vi "Read Enabled Values.vi"(8 "error in (no error)":errorcluster, 11 "No-Op in":refnum<class "No-Op Output.lvclass">) -> (0 "error out":errorcluster, 1 "Data Values Native":dbl[](array[numeric]), 2 "Data Values Engineering":dbl[](array[numeric]), 3 "No-Op out":refnum<class "No-Op Output.lvclass">)   [LabVIEW 2018, in "No-Op Output.lvclass"]
uses:
  No-Op Output.lvclass
  No-Op Output.lvclass/No-Op Output.ctl
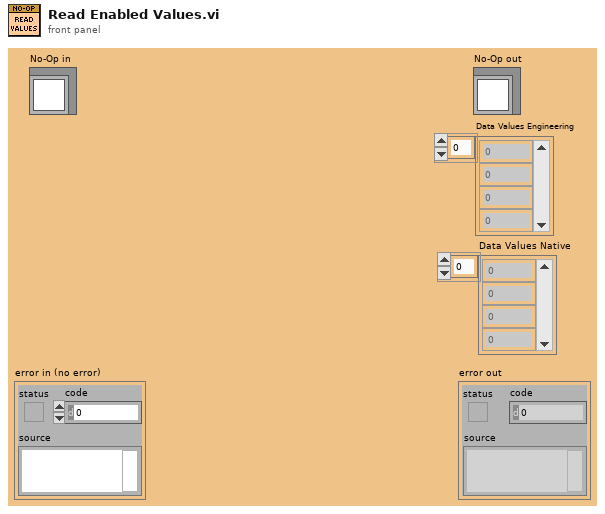
[diagram p1: front panel]
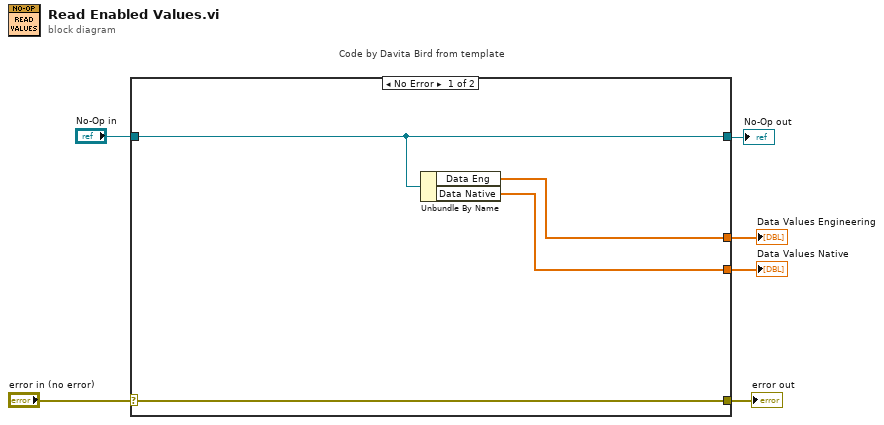
[diagram p0: block diagram]
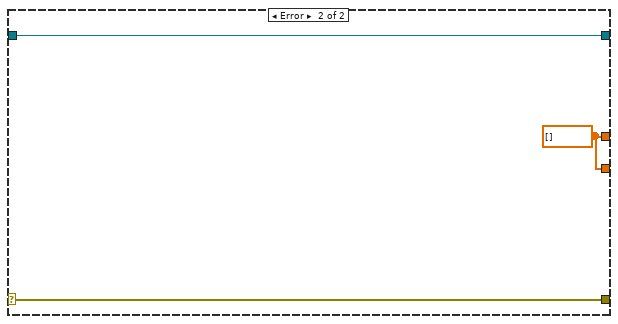
[diagram p2: hidden frame]
diagram:
  n1 = case "Code by Davita Bird from template" shown="No Error" "error in (no error)" {
    selector: "error in (no error)" -> [w10 w13]
    tunnel: [w10 w13] -> w5
    tunnel: [w9 w12] -> w2
    tunnel: "No-Op in" -> [w9 w12]
    tunnel: [w8 w11] -> w4
    tunnel: [w7 w11] -> w1
    frame No Error {
      n2 = Unbundle By Name(w9) -> ("Data Eng"=w8:dbl[], "Data Native"=w7:dbl[])
    }
    frame Error {
      w11 = dbl[] [] ("array type (2D Dbl)")
    }
  }
  "error out" <- w5
  "Data Values Engineering" <- w4
  "No-Op out" <- w2
  "Data Values Native" <- w1
